vi "State Machine.vi"(8 "error in (no error)":errorcluster) -> (0 "error out":errorcluster)   [LabVIEW 2018]
uses:
  State Machine/State Machine.lvclass
  State Machine/State Machine.lvclass/State Machine.ctl
  <vilib>/addons/_JKI Toolkits/Caraya/classes/Test/Test.lvclass
  <vilib>/addons/_JKI Toolkits/Caraya/classes/Assert/Assert.lvclass
panel:
  in  "State Machine.lvclass":refnum<class "State Machine.lvclass">
  in  "State Machine in 2":refnum<class "State Machine.lvclass">
  in  "State Machine in":refnum<class "State Machine.lvclass">
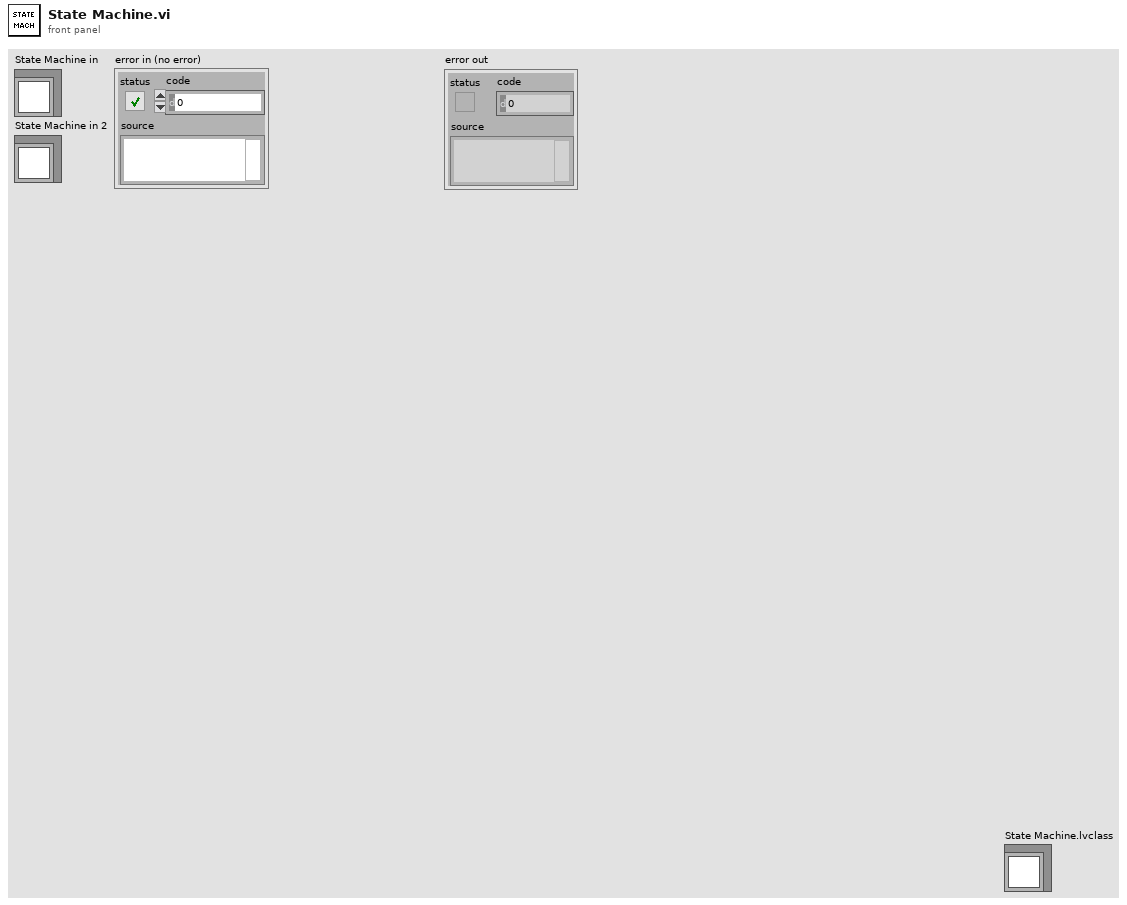
[diagram p1: front panel]
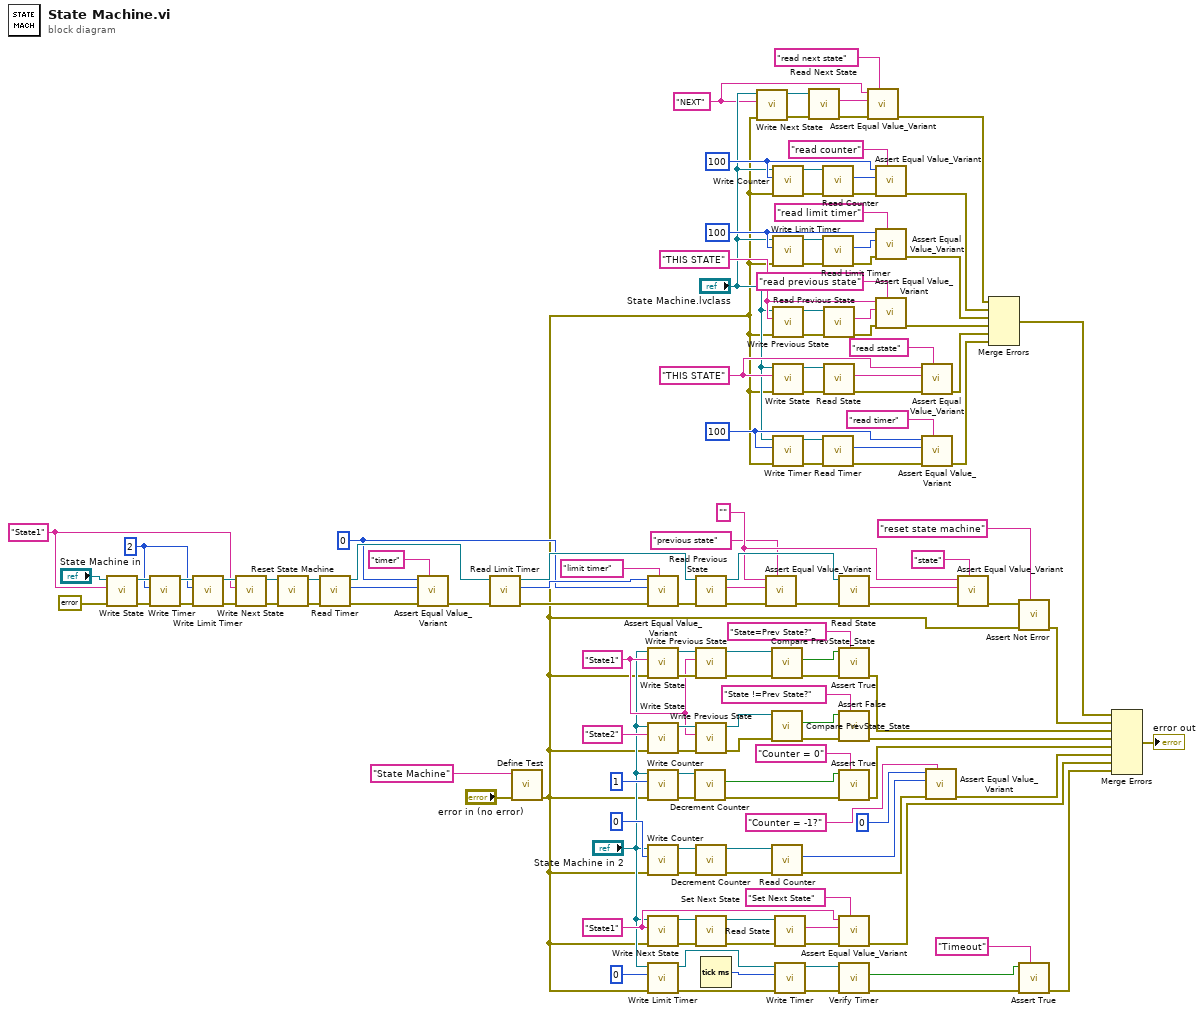
[diagram p0: block diagram]
diagram:
  w4 = "NEXT" ("Next State")
  w11 = 100
  w19 = "THIS STATE" ("Previous State")
  w27 = "THIS STATE" ("Previous State")
  w33 = 100
  w32 = 100
  w64 = "State1" ("Label (VI Title)")
  w73 = "" ("State")
  w80 = u16 0 ("Counter")
  w96 = u16 2 ("Counter")
  w97 = "State1" ("Label (VI Title)")
  w121 = "State1" ("Label (VI Title)")
  n1 = call-dynamic "Write State.vi"("error in (no error)"=errorcluster {"status"=FALSE, "code"=0, "source"=""}, "State"=w97, "State Machine in"="State Machine in") -> ("error out"=w101:errorcluster, "State Machine out"=w100:refnum<class "State Machine.lvclass">)  [unwired: 7 in]
  n2 = call "Write Timer.vi"("error in (no error)"=w101, "Timer"=w96, "State Machine in"=w100) -> ("error out"=w102:errorcluster, "State Machine out"=w99:refnum<class "State Machine.lvclass">)  [unwired: 7 in]
  n3 = call "Write Limit Timer.vi"("error in (no error)"=w102, "Limit Timer"=w96, "State Machine in"=w99) -> ("error out"=w103:errorcluster, "State Machine out"=w98:refnum<class "State Machine.lvclass">)  [unwired: 7 in]
  n4 = call "Write Next State.vi"("error in (no error)"=w103, "Next State"=w97, "State Machine in"=w98) -> ("error out"=w95:errorcluster, "State Machine out"=w94:refnum<class "State Machine.lvclass">)  [unwired: 7 in]
  n5 = call "Reset State Machine.vi"("error in (no error)"=w95, "State Machine in"=w94) -> ("error out"=w89:errorcluster, "State Machine out"=w90:refnum<class "State Machine.lvclass">)  [unwired: 8 in]
  n6 = call "Read Timer.vi"("error in (no error)"=w89, "State Machine in"=w90) -> ("error out"=w88:errorcluster, "Timer"=w86:u32, "State Machine out"=w91:refnum<class "State Machine.lvclass">)  [unwired: 7 in]
  n7 = call <vilib>:"Assert Equal Value_Variant.vi"("Label"="timer", "error in (no error)"=w88, "Actual"=w86, "Expected"=w80) -> ("error out"=w87:errorcluster)  [unwired: 6 in, 1 out]
  n8 = call "Read Limit Timer.vi"("error in (no error)"=w87, "State Machine in"=w91) -> ("error out"=w82:errorcluster, "Limit Timer"=w81:u32, "State Machine out"=w92:refnum<class "State Machine.lvclass">)  [unwired: 7 in]
  n9 = call <vilib>:"Define Test.vi"("error in (no error)"="error in (no error)", "Label (VI Title)"="State Machine") -> ("error out"=w1:errorcluster)  [unwired: 8 in, 1 out]
  n10 = call <vilib>:"Assert Equal Value_Variant.vi"("Label"="limit timer", "error in (no error)"=w82, "Actual"=w80, "Expected"=w81) -> ("error out"=w83:errorcluster)  [unwired: 6 in, 1 out]
  n11 = call-dynamic "Write State.vi"("error in (no error)"=w1, "State"=w121, "State Machine in"="State Machine in 2") -> ("error out"=w137:errorcluster, "State Machine out"=w136:refnum<class "State Machine.lvclass">)  [unwired: 7 in]
  n12 = call-dynamic "Write State.vi"("error in (no error)"=w1, "State"="State2" ("Label (VI Title)"), "State Machine in"="State Machine in 2") -> ("error out"=w123:errorcluster, "State Machine out"=w124:refnum<class "State Machine.lvclass">)  [unwired: 7 in]
  n13 = call "Write Counter.vi"("error in (no error)"=w1, "Counter"=u16 1, "State Machine in"="State Machine in 2") -> ("error out"=w118:errorcluster, "State Machine out"=w117:refnum<class "State Machine.lvclass">)  [unwired: 7 in]
  n14 = call "Write Counter.vi"("error in (no error)"=w1, "Counter"=u16 0, "State Machine in"="State Machine in 2") -> ("error out"=w111:errorcluster, "State Machine out"=w112:refnum<class "State Machine.lvclass">)  [unwired: 7 in]
  n15 = call "Write Next State.vi"("error in (no error)"=w1, "Next State"=w64, "State Machine in"="State Machine in 2") -> ("error out"=w71:errorcluster, "State Machine out"=w70:refnum<class "State Machine.lvclass">)  [unwired: 7 in]
  n16 = call "Write Limit Timer.vi"("error in (no error)"=w1, "Limit Timer"=u32 0, "State Machine in"="State Machine in 2") -> ("error out"=w53:errorcluster, "State Machine out"=w52:refnum<class "State Machine.lvclass">)  [unwired: 7 in]
  n17 = call "Decrement Counter.vi"("error in (no error)"=w118, "State Machine in"=w117) -> ("error out"=w116:errorcluster, "counter = zero"=w113:bool)  [unwired: 7 in, 1 out]
  n18 = call-dynamic "Read Previous State.vi"("error in (no error)"=w83, "State Machine in"=w92) -> ("error out"=w79:errorcluster, "Previous State"=w74:string, "State Machine out"=w93:refnum<class "State Machine.lvclass">)  [unwired: 7 in]
  n19 = call-dynamic "Write Previous State.vi"("error in (no error)"=w137, "Previous State"=w121, "State Machine in"=w136) -> ("error out"=w138:errorcluster, "State Machine out"=w135:refnum<class "State Machine.lvclass">)  [unwired: 7 in]
  n20 = call-dynamic "Write Previous State.vi"("error in (no error)"=w123, "Previous State"=w121, "State Machine in"=w124) -> ("error out"=w122:errorcluster, "State Machine out"=w125:refnum<class "State Machine.lvclass">)  [unwired: 7 in]
  n21 = call "Decrement Counter.vi"("error in (no error)"=w111, "State Machine in"=w112) -> ("error out"=w109:errorcluster, "State Machine out"=w108:refnum<class "State Machine.lvclass">)  [unwired: 7 in, 1 out]
  n22 = call "Set Next State.vi"("error in (no error)"=w71, "State Machine in"=w70) -> ("error out"=w68:errorcluster, "State Machine out"=w67:refnum<class "State Machine.lvclass">)  [unwired: 8 in]
  n23 = Tick Count (ms)() -> (millisecond timer value=w51:u32)
  n24 = call "Write Next State.vi"("error in (no error)"=w1, "Next State"=w4, "State Machine in"="State Machine.lvclass") -> ("error out"=w8:errorcluster, "State Machine out"=w6:refnum<class "State Machine.lvclass">)  [unwired: 7 in]
  n25 = call <vilib>:"Assert Equal Value_Variant.vi"("Label"="previous state", "error in (no error)"=w79, "Actual"=w74, "Expected"=w73) -> ("error out"=w78:errorcluster)  [unwired: 6 in, 1 out]
  n26 = call "Compare PrevState_State.vi"("error in (no error)"=w138, "State Machine in"=w135) -> ("error out"=w133:errorcluster, "prev = state ?"=w131:bool)  [unwired: 7 in, 1 out]
  n27 = call "Compare PrevState_State.vi"("error in (no error)"=w122, "State Machine in"=w125) -> ("error out"=w126:errorcluster, "prev = state ?"=w128:bool)  [unwired: 7 in, 1 out]
  n28 = call "Read Counter.vi"("error in (no error)"=w109, "State Machine in"=w108) -> ("error out"=w106:errorcluster, "Counter"=w50:u16)  [unwired: 7 in, 1 out]
  n29 = call "Write Counter.vi"("error in (no error)"=w1, "Counter"=w33, "State Machine in"="State Machine.lvclass") -> ("error out"=w44:errorcluster, "State Machine out"=w45:refnum<class "State Machine.lvclass">)  [unwired: 7 in]
  n30 = call "Write Limit Timer.vi"("error in (no error)"=w1, "Limit Timer"=w32, "State Machine in"="State Machine.lvclass") -> ("error out"=w37:errorcluster, "State Machine out"=w34:refnum<class "State Machine.lvclass">)  [unwired: 7 in]
  n31 = call-dynamic "Write Previous State.vi"("error in (no error)"=w1, "Previous State"=w27, "State Machine in"="State Machine.lvclass") -> ("error out"=w30:errorcluster, "State Machine out"=w29:refnum<class "State Machine.lvclass">)  [unwired: 7 in]
  n32 = call-dynamic "Write State.vi"("error in (no error)"=w1, "State"=w19, "State Machine in"="State Machine.lvclass") -> ("error out"=w23:errorcluster, "State Machine out"=w22:refnum<class "State Machine.lvclass">)  [unwired: 7 in]
  n33 = call "Write Timer.vi"("error in (no error)"=w1, "Timer"=w11, "State Machine in"="State Machine.lvclass") -> ("error out"=w14:errorcluster, "State Machine out"=w13:refnum<class "State Machine.lvclass">)  [unwired: 7 in]
  n34 = call-dynamic "Read State.vi"("error in (no error)"=w68, "State Machine in"=w67) -> ("error out"=w66:errorcluster, "State"=w65:string)  [unwired: 7 in, 1 out]
  n35 = call "Write Timer.vi"("error in (no error)"=w53, "Timer"=w51, "State Machine in"=w52) -> ("error out"=w55:errorcluster, "State Machine out"=w54:refnum<class "State Machine.lvclass">)  [unwired: 7 in]
  n36 = call-dynamic "Read Next State.vi"("error in (no error)"=w8, "State Machine in"=w6) -> ("error out"=w9:errorcluster, "Next State"=w5:string)  [unwired: 7 in, 1 out]
  n37 = call "Read Counter.vi"("error in (no error)"=w44, "State Machine in"=w45) -> ("error out"=w43:errorcluster, "Counter"=w42:u16)  [unwired: 7 in, 1 out]
  n38 = call "Read Limit Timer.vi"("error in (no error)"=w37, "State Machine in"=w34) -> ("error out"=w38:errorcluster, "Limit Timer"=w36:u32)  [unwired: 7 in, 1 out]
  n39 = call "Read Timer.vi"("error in (no error)"=w14, "State Machine in"=w13) -> ("error out"=w15:errorcluster, "Timer"=w12:u32)  [unwired: 7 in, 1 out]
  n40 = call-dynamic "Read Previous State.vi"("error in (no error)"=w30, "State Machine in"=w29) -> ("error out"=w31:errorcluster, "Previous State"=w28:string)  [unwired: 7 in, 1 out]
  n41 = call-dynamic "Read State.vi"("error in (no error)"=w23, "State Machine in"=w22) -> ("error out"=w21:errorcluster, "State"=w20:string)  [unwired: 7 in, 1 out]
  n42 = call-dynamic "Read State.vi"("error in (no error)"=w78, "State Machine in"=w93) -> ("error out"=w77:errorcluster, "State"=w75:string)  [unwired: 7 in, 1 out]
  n43 = call <vilib>:"Assert True.vi"("Label"="State=Prev State?", "error in (no error)"=w133, "True?"=w131) -> ("error out"=w132:errorcluster)  [unwired: 7 in, 1 out]
  n44 = call <vilib>:"Assert False.vi"("Label"="State !=Prev State?", "error in (no error)"=w126, "False?"=w128) -> ("error out"=w120:errorcluster)  [unwired: 7 in, 1 out]
  n45 = call <vilib>:"Assert True.vi"("Label"="Counter = 0", "error in (no error)"=w116, "True?"=w113) -> ("error out"=w114:errorcluster)  [unwired: 7 in, 1 out]
  n46 = call <vilib>:"Assert Equal Value_Variant.vi"("Label"="Set Next State", "error in (no error)"=w66, "Actual"=w65, "Expected"=w64) -> ("error out"=w62:errorcluster)  [unwired: 6 in, 1 out]
  n47 = call "Verify Timer.vi"("error in (no error)"=w55, "State Machine in"=w54) -> ("error out"=w59:errorcluster, "time out"=w56:bool)  [unwired: 7 in, 1 out]
  n48 = call <vilib>:"Assert Equal Value_Variant.vi"("Label"="read next state", "error in (no error)"=w9, "Actual"=w5, "Expected"=w4) -> ("error out"=w2:errorcluster)  [unwired: 6 in, 1 out]
  n49 = call <vilib>:"Assert Equal Value_Variant.vi"("Label"="read counter", "error in (no error)"=w43, "Actual"=w42, "Expected"=w33) -> ("error out"=w40:errorcluster)  [unwired: 6 in, 1 out]
  n50 = call <vilib>:"Assert Equal Value_Variant.vi"("Label"="read limit timer", "error in (no error)"=w38, "Actual"=w36, "Expected"=w32) -> ("error out"=w39:errorcluster)  [unwired: 6 in, 1 out]
  n51 = call <vilib>:"Assert Equal Value_Variant.vi"("Label"="read previous state", "error in (no error)"=w31, "Actual"=w28, "Expected"=w27) -> ("error out"=w25:errorcluster)  [unwired: 6 in, 1 out]
  n52 = call <vilib>:"Assert Equal Value_Variant.vi"("Label"="read state", "error in (no error)"=w21, "Actual"=w20, "Expected"=w19) -> ("error out"=w24:errorcluster)  [unwired: 6 in, 1 out]
  n53 = call <vilib>:"Assert Equal Value_Variant.vi"("Label"="read timer", "error in (no error)"=w15, "Actual"=w12, "Expected"=w11) -> ("error out"=w17:errorcluster)  [unwired: 6 in, 1 out]
  n54 = call <vilib>:"Assert Equal Value_Variant.vi"("Label"="Counter = -1?", "error in (no error)"=w106, "Actual"=w50, "Expected"=u16 0 ("Counter")) -> ("error out"=w105:errorcluster)  [unwired: 6 in, 1 out]
  n55 = call <vilib>:"Assert Equal Value_Variant.vi"("Label"="state", "error in (no error)"=w77, "Actual"=w75, "Expected"=w73) -> ("error out"=w76:errorcluster)  [unwired: 6 in, 1 out]
  n56 = Merge Errors(w2, w40, w39, w25, w24, w17) -> (w10:errorcluster)
  n57 = call <vilib>:"Assert Not Error.vi"("Label"="reset state machine", "error in (no error)"=w1, "Not Error?"=w76) -> ("error out"=w85:errorcluster)  [unwired: 7 in, 1 out]
  n58 = call <vilib>:"Assert True.vi"("Label"="Timeout", "error in (no error)"=w59, "True?"=w56) -> ("error out"=w58:errorcluster)  [unwired: 7 in, 1 out]
  n59 = Merge Errors(w10, w85, w132, w120, w114, w105, w62, w58) -> (→"error out":errorcluster)
